vi "ziModGetNodeValueInteger.vi"(0 "ModHandle In":T1 {"ModHandle" format="0x%08x"; "Conn" format="0x%08x"}, 7 "Path":string, 11 "error in":errorcluster) -> (4 "ModHandle Out":T1 {"ModHandle" format="0x%08x"; "Conn" format="0x%08x"}, 8 "Value":i64, 15 "error out":errorcluster)   [LabVIEW 2009, in "Zurich Instruments LabOne.lvlib"]
doc: "FOR MODULES This vi retrieves the numerical value of the specified node as an int64-type value. The vi returns the value first found that matches Path if more than one value is available (a wildcard is used in the Path)."
uses:
  <instrlib>/Zurich Instruments LabOne/Zurich Instruments LabOne.lvlib
  <instrlib>/Zurich Instruments LabOne/Public/Modules/ziTypeModHandle.ctl
  <instrlib>/Zurich Instruments LabOne/Private/ziLV32.dll
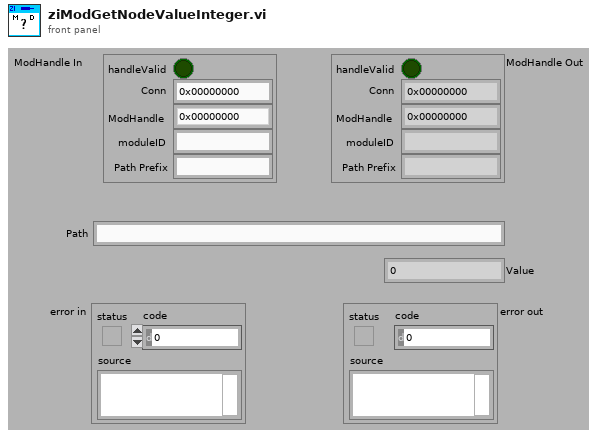
[diagram p1: front panel]
types:
  T1 = typedef "Zurich Instruments LabOne.lvlib/ziTypeModHandle.ctl" = cluster{"handleValid":bool, "Conn":u64, "ModHandle":u64, "moduleID":string, "Path Prefix":string}
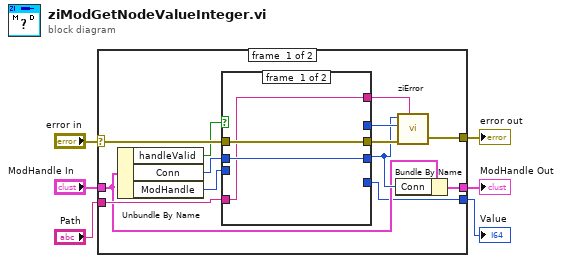
[diagram p0: block diagram]
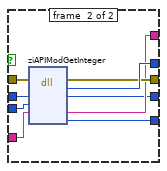
[diagram p2: hidden frame]
diagram:
  n1 = case shown="No Error" "error in" {
    selector: "error in" -> [w15 w33]
    tunnel: [w17 w33] -> w6
    tunnel: [w16 w32] -> w2
    tunnel: "ModHandle In" -> [w10 w32]
    tunnel: "Path" -> [w11 _]
    tunnel: [w7 _] -> w1
    frame #0 {
      n2 = Unbundle By Name(w10) -> ("handleValid"=w8:bool, "Conn"=w13:u64, "ModHandle"=w9:u64)
      n3 = case shown="True" w8 {
        tunnel: [_ w31] -> w19
        tunnel: [w22 w30] -> w18
        tunnel: w15 -> [w22 w29]
        tunnel: [w20 w28] -> w14
        tunnel: w13 -> [w21 w27]
        tunnel: [w21 w26] -> w12
        tunnel: w11 -> [w20 w25]
        tunnel: w9 -> [_ w24]
        tunnel: [_ w23] -> w7
        frame #0 {
        }
        frame #1 {
          n4 = dll-call lib="C:/Program Files (x86)/National Instruments/LabVIEW 2009/instr.lib/Zurich Instruments LabOne/Private/ziLV*.*" fn="ziAPIModGetInteger" label="ziAPIModGetString"(error in=w29, "Conn"=w27, "ModHandle"=w24, "Path"=w25) -> (error out=w30:errorcluster, "return type"=w31:u32, "Conn"=w26:u64, "Path"=w28:string, "Value"=w23:i64)  [unwired: 3 in, 2 out]
        }
      }
      n5 = Bundle By Name(cluster=w10, "Conn"=w12) -> (w16:T1)
      n6 = call <instrlib>:"ziError.vi"("Conn"=w12, "ziErrorCode"=w19, "Error In"=w18, "Annotation"=w14) -> ("Error Out"=w17:errorcluster)  [unwired: 2 in]
    }
    frame #1 {
    }
  }
  "error out" <- w6
  "Value" <- w1
  "ModHandle Out" <- w2
